vi "Motor Speed AO Message Loop.vi"(8 "error in (no error)":errorcluster, 11 "Message Queues":T1) -> (0 "error out":errorcluster)   [LabVIEW 2016, in "Motor Speed AO.lvlib"]
doc: "The message loop subVI to handle messages pertaining to logging data."
uses:
  Motor Speed AO.lvlib
  support/Message Queue/All Message Queues.ctl
  support/Message Queue/Message Cluster.ctl
  MSpeed AO State.ctl
  MSpeed_MHL Data.ctl
  MSpeed AO HW Config.ctl
  <vilib>/DAQmx/write.llb/DAQmx Write (Analog Wfm 1Chan NSamp).vi
  support/Message Queue/Enqueue Message (Single).vi
  <vilib>/DAQmx/create/channels.llb/DAQmx Create Channel (AO-Voltage-Basic).vi
  <vilib>/DAQmx/configure/timing.llb/DAQmx Timing (Sample Clock).vi
  <vilib>/DAQmx/miscellaneous.llb/DAQmx Fill In Error Info.vi
  <vilib>/Utility/error.llb/Error Cluster From Error Code.vi
  <vilib>/ErrorRing/Error Ring.xnode
  support/Message Queue/Message Queue.lvlib
  <resource>/objmgr/daqmx.rc
  <vilib>/measure/NI_MABase.lvlib
  <instrlib>/Pololu Motor Controller/Pololu Motor Controller.lvlib
panel:
  out "Actual Sample Rate":dbl=1000.0 format="%0.2f"
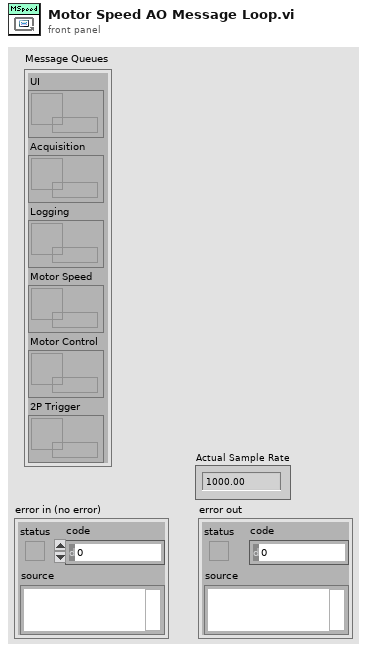
[diagram p1: front panel]
types:
  T1 = typedef "Message Queue.lvlib/All Message Queues.ctl" = cluster{"UI":refnum<queue>, "Acquisition":refnum<queue>, "Logging":refnum<queue>, "Motor Speed":refnum<queue>, "Motor Control":refnum<queue>, "2P Trigger":refnum<queue>}
  T2 = typedef "Motor Speed AO.lvlib/MSpeed AO State.ctl" = enum16{"Idle", "Running"}
  T3 = enum16{"Sine Wave", "Triangle Wave", "Square Wave", "Sawtooth Wave"}
  T4 = typedef "Motor Speed AO.lvlib/MSpeed_MHL Data.ctl" = cluster{"MSpeed HW Config":T5, "Motor VISA resource name":refnum<visa-resource-name>}
  T5 = typedef "Motor Speed AO.lvlib/MSpeed AO HW Config.ctl" = cluster{"MSpeed AO Channel":tag, "Sample Rate(Hz)":dbl, "MSpeed AO Task":refnum<k21>}
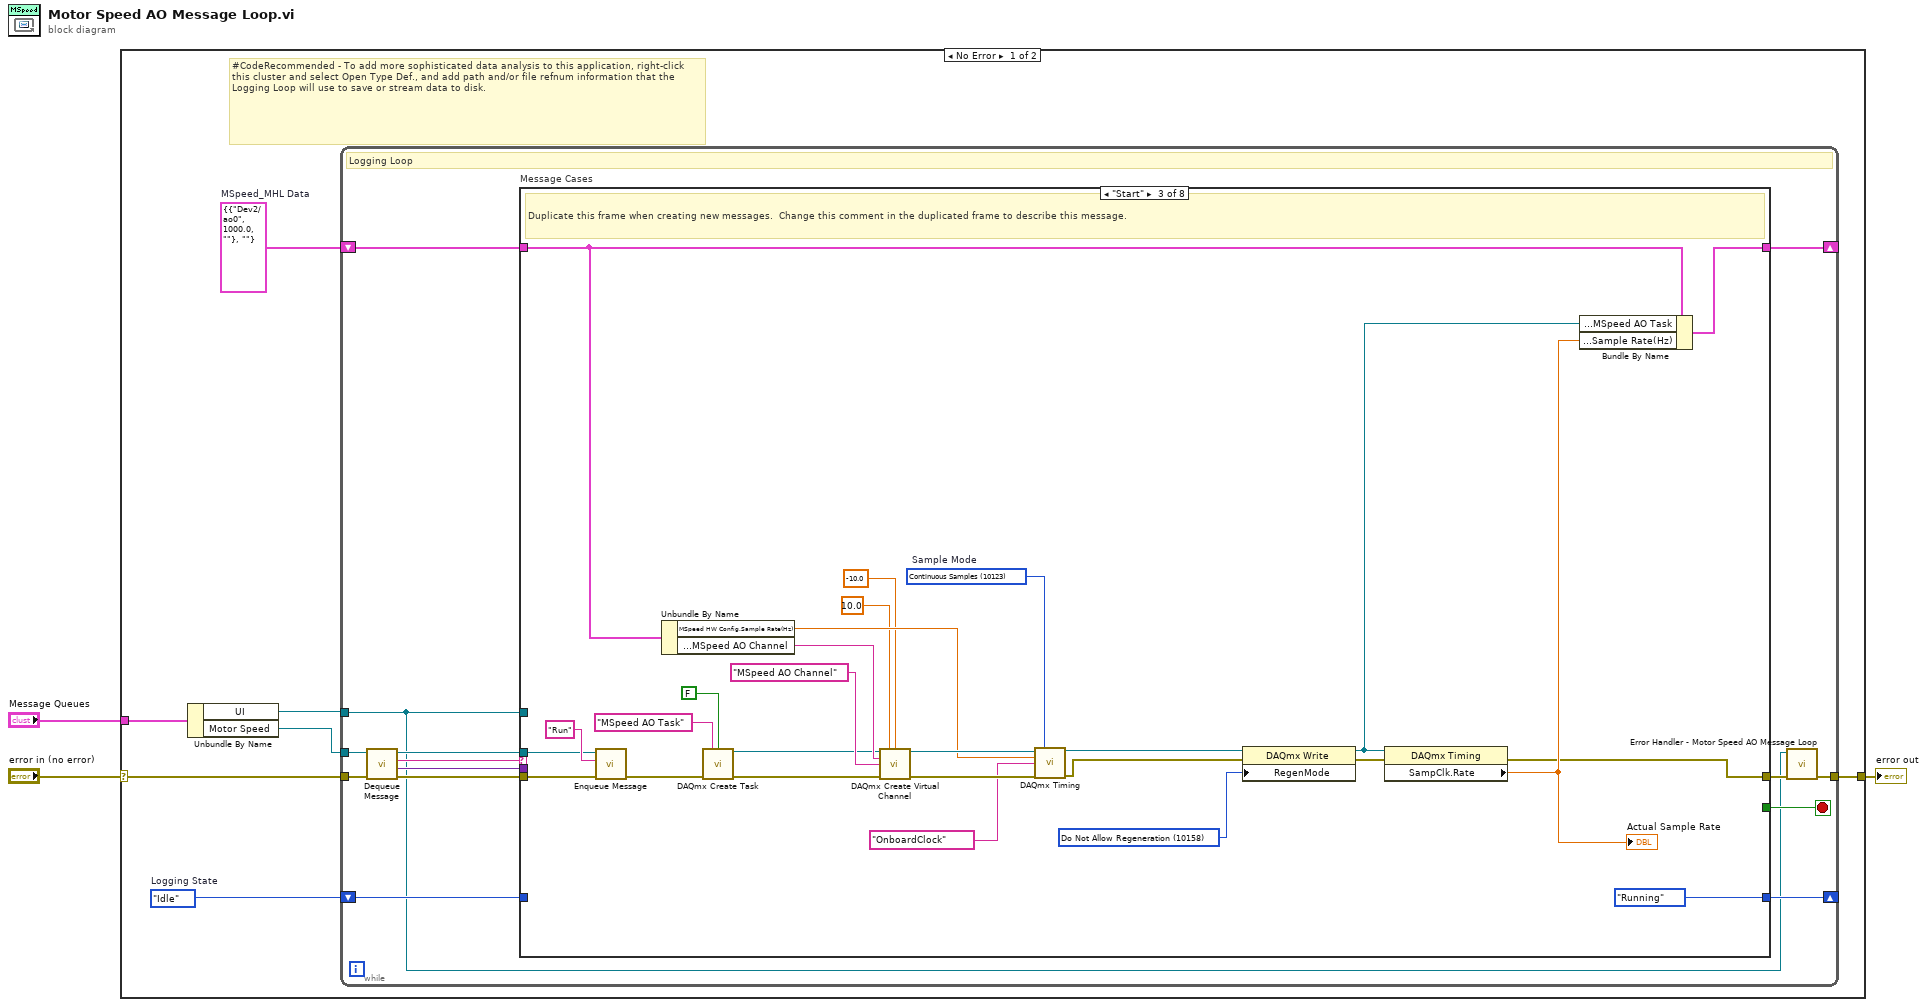
[diagram p0: block diagram]
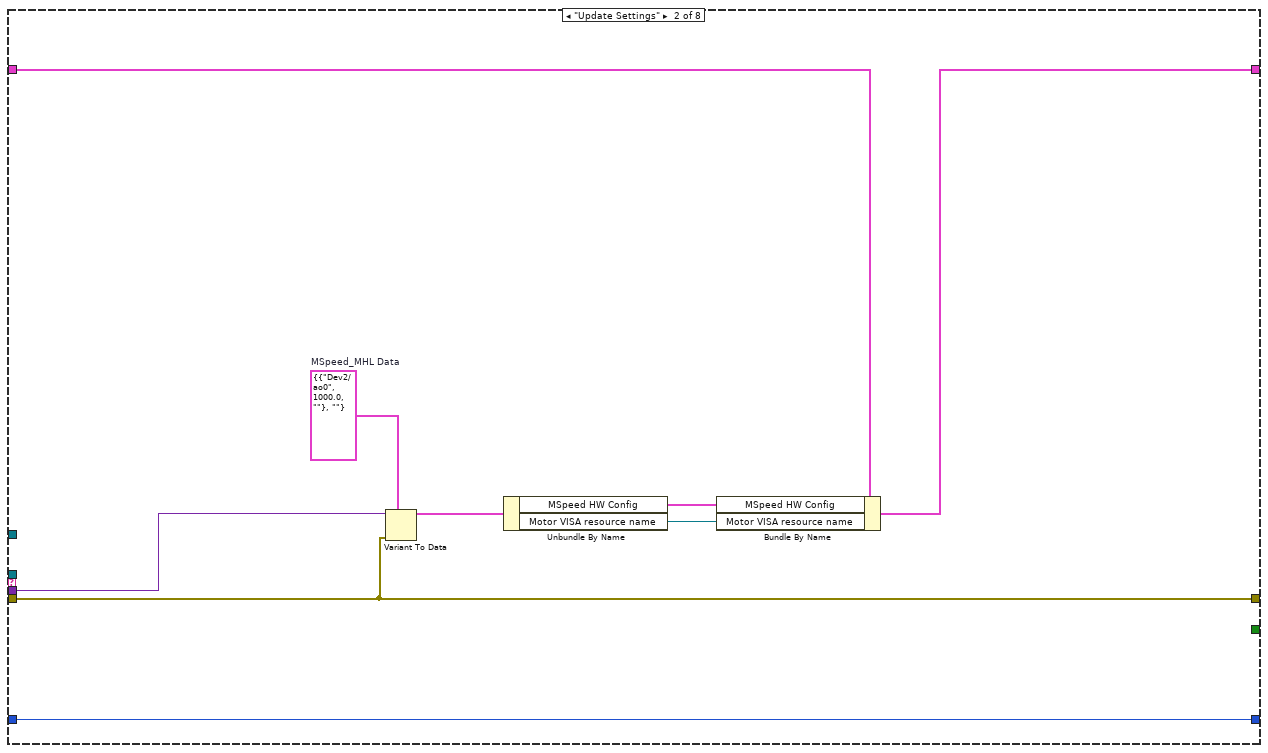
[diagram p3: hidden frame]
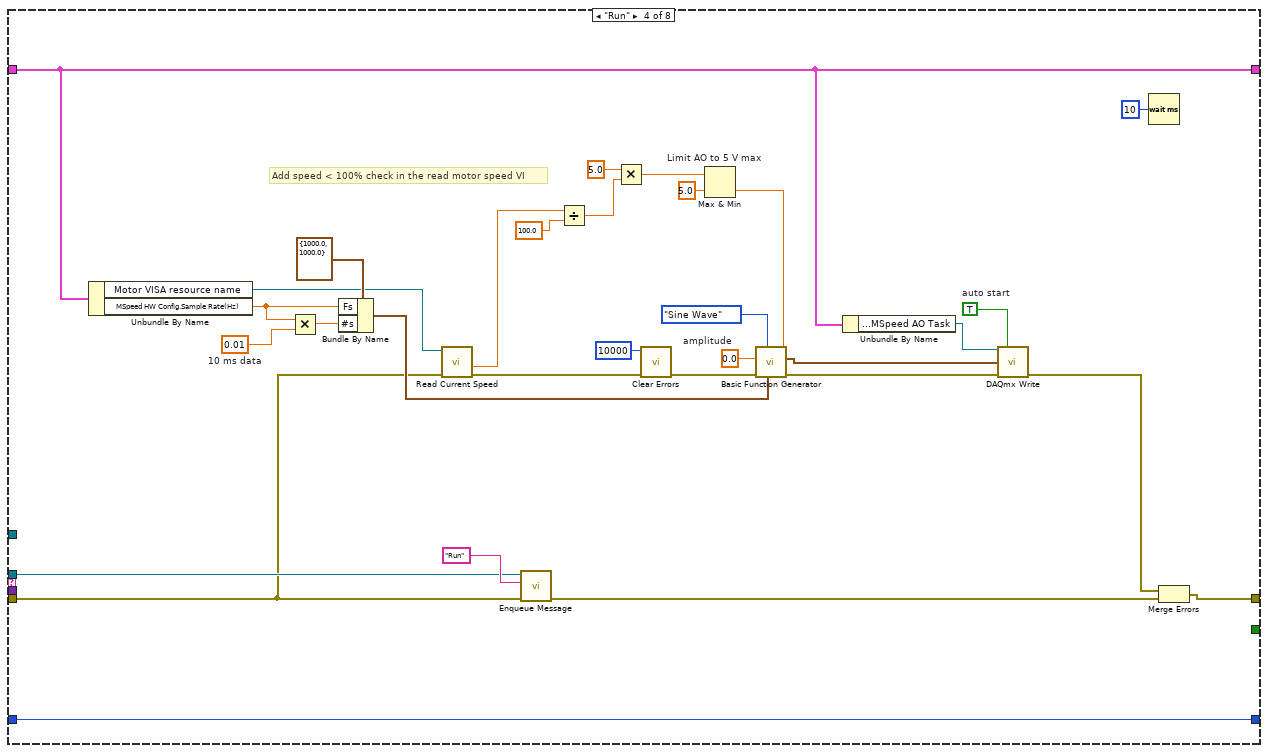
[diagram p4: hidden frame]
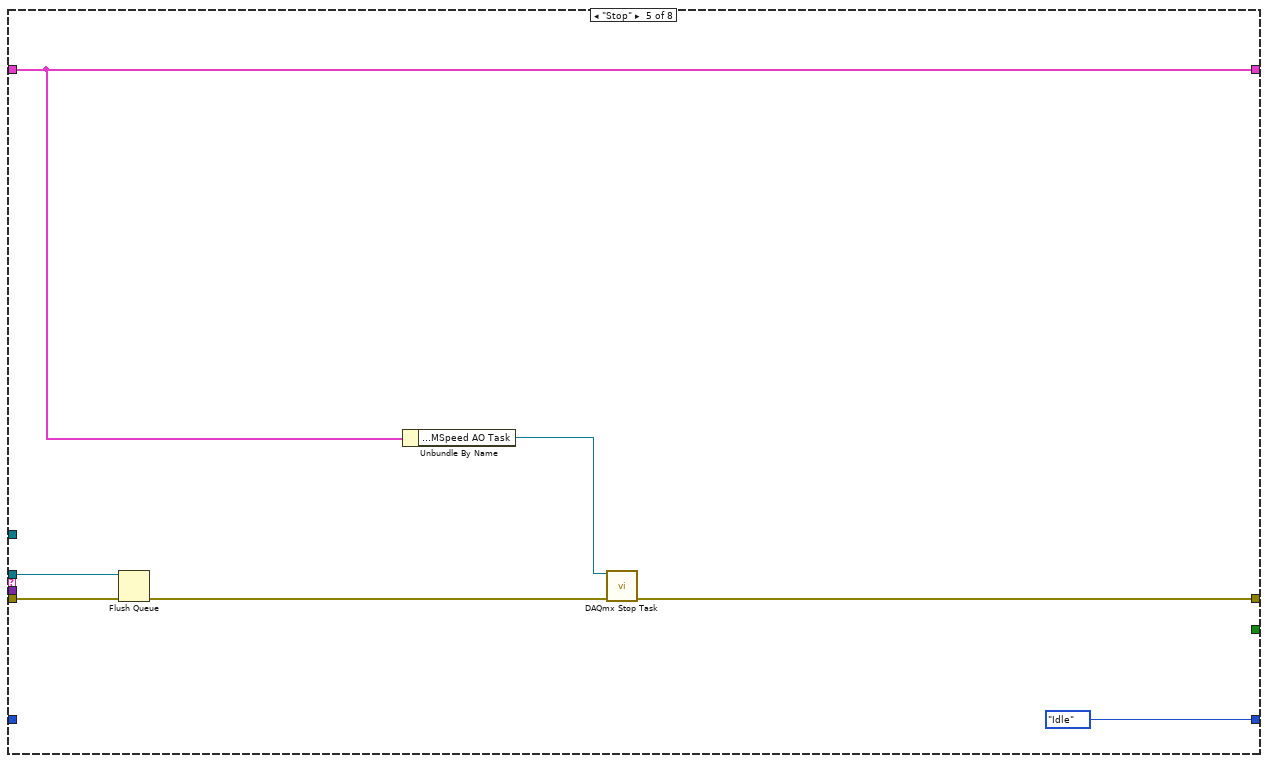
[diagram p5: hidden frame]
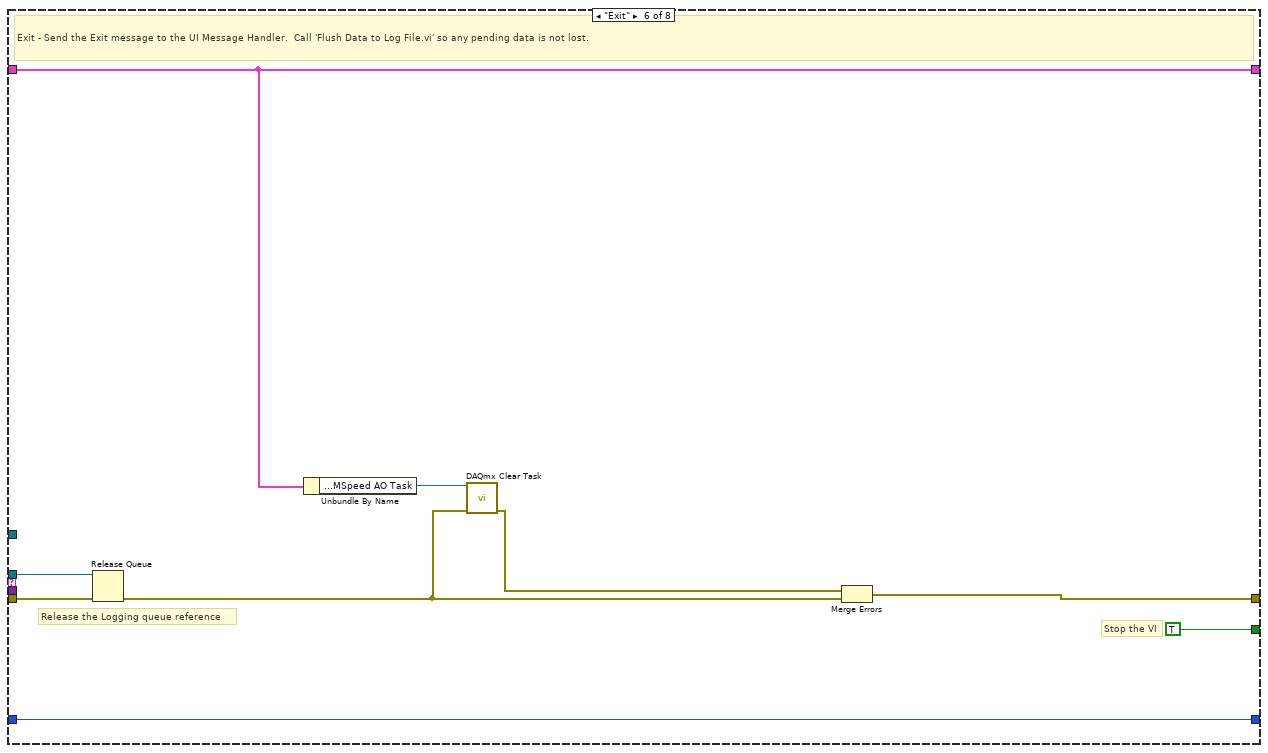
[diagram p6: hidden frame]
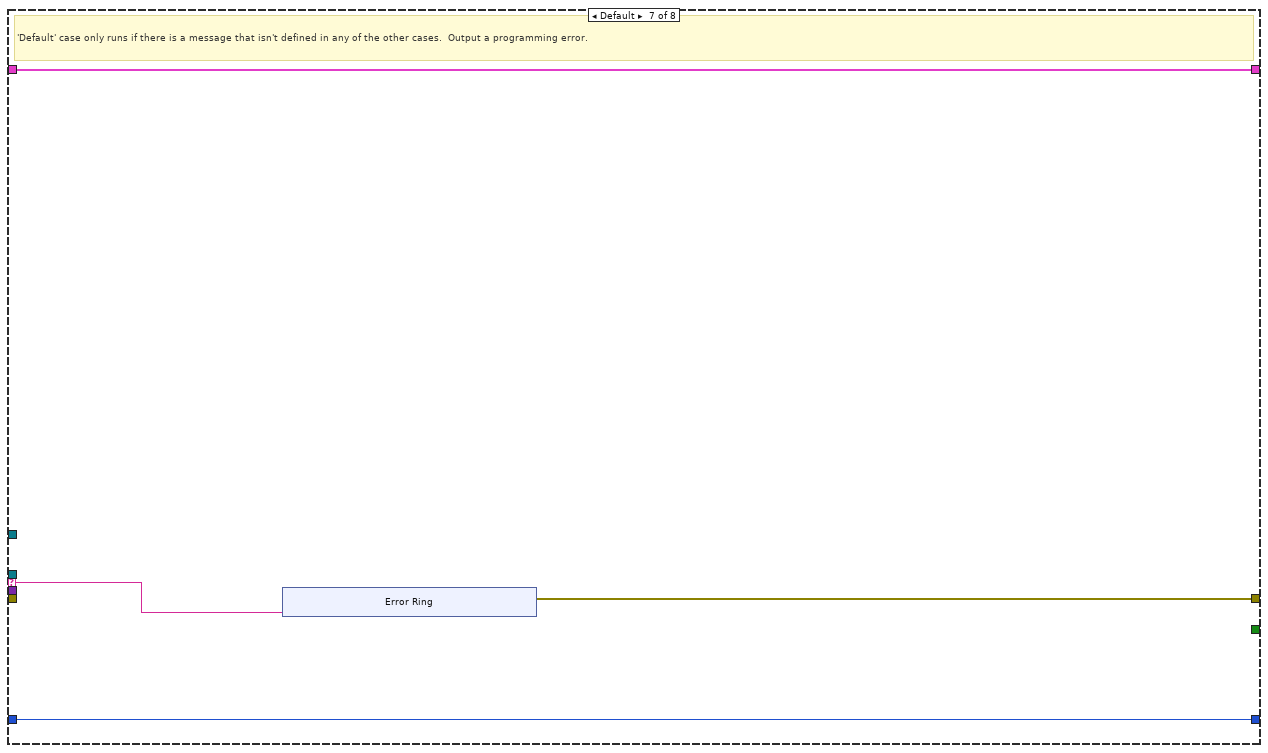
[diagram p7: hidden frame]
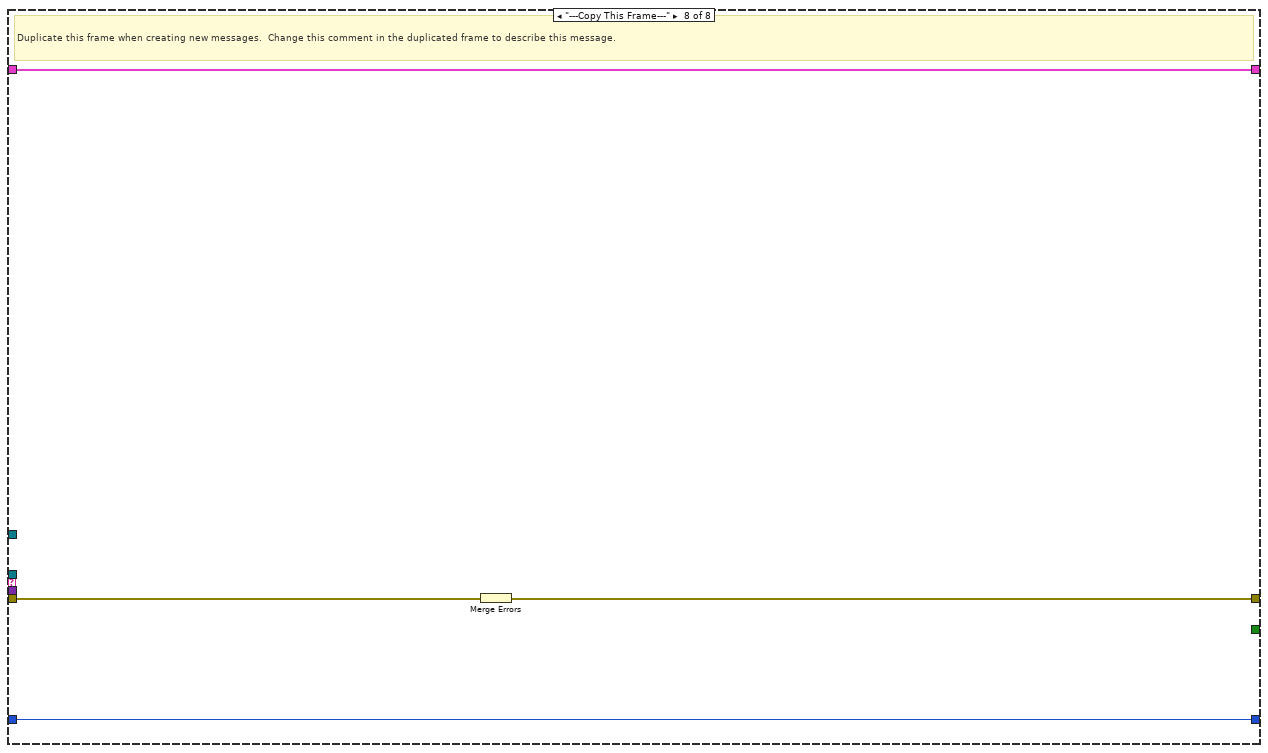
[diagram p8: hidden frame]
diagram:
  n1 = case shown="No Error" "error in (no error)" {
    selector: "error in (no error)" -> [w7 w126]
    tunnel: "Message Queues" -> [w10 _]
    tunnel: [w8 w126] -> w2
    frame No Error {
      w4 = T4 {"MSpeed HW Config"={"MSpeed AO Channel"="Dev2/ao0", "Sample Rate(Hz)"=1000.0, "MSpeed AO Task"=""}, "Motor VISA resource name"=""}  # MSpeed_MHL Data
      w5 = MSpeed_AO_State."Idle"  # Logging State
      # "#CodeRecommended - To add more sophisticated data analysis to this application, right-click this cluster and select Open Type Def., and add path and/or file refnum information that the Logging Loop will use to save or stream data to disk."
      n2 = Unbundle By Name(w10) -> ("UI"=w6:refnum<queue>, "Motor Speed"=w9:refnum<queue>)
      n3 = while {
        tunnel: w9 -> [w16]
        shift-right: [w23] -> _
        shift-left: w4 -> [w24]
        tunnel: w6 -> [w11]
        shift-right: [w14] -> _
        shift-left: w5 -> [w15]
        tunnel: w7 -> [w21]
        tunnel: [w13] -> w8
        stop <- w22 stop-if-true
        # "Logging Loop"
        n4 = call "Dequeue Message.vi"("error in (no error)"=w21, "Message Queue"=w16) -> ("error out"=w20:errorcluster, "Message Data"=w18:variant, "Message"=w19:string, "dup Message Queue"=w17:refnum<queue>)  [unwired: 6 in]
        n5 = case "Message Cases" shown="\"Start\"" w19 {
          selector: w19 -> [_ _ _ _ _ _ w111 _]
          tunnel: w17 -> [_ _ w61 w80 w96 w107 _ _]
          tunnel: w20 -> [w26 w35 w57 w75 w98 w108 _ w125]
          tunnel: [w26 w35 w37 w79 w101 w109 w112 w123] -> w12
          tunnel: w24 -> [w27 w33 w53 w86 w100 w103 w114 w124]
          tunnel: [w27 w32 w50 w86 w100 w103 w114 w124] -> w23
          tunnel: [_ _ _ _ _ TRUE _ _] -> w22
          tunnel: w18 -> [_ w34 _ _ _ _ _ _]
          tunnel: w11 -> [_ _ _ _ _ _ _ _]
          tunnel: w15 -> [w25 w36 _ w94 _ w106 w113 w122]
          tunnel: [w25 w36 MSpeed_AO_State."Running" ("Logging State") w94 MSpeed_AO_State."Idle" ("Logging State") w106 w113 w122] -> w14
          frame "Initialize" {
            # "Initialize - gets called when first launched. Currently a no-op."
          }
          frame "Update Settings" {
            w28 = T4 {"MSpeed HW Config"={"MSpeed AO Channel"="Dev2/ao0", "Sample Rate(Hz)"=1000.0, "MSpeed AO Task"=""}, "Motor VISA resource name"=""}  # MSpeed_MHL Data
            n6 = Variant To Data(error in=w35, type=w28, Variant=w34) -> (data=w29:T4)  [unwired: 1 out]
            n7 = Unbundle By Name(w29) -> ("MSpeed HW Config"=w30:T5, "Motor VISA resource name"=w31:refnum<visa-resource-name>)
            n8 = Bundle By Name(cluster=w33, "MSpeed HW Config"=w30, "Motor VISA resource name"=w31) -> (w32:T4)
          }
          frame "Start" {
            w55 = 10158 items=["Allow Regeneration"=10097, "Do Not Allow Regeneration"=10158] ("RegenMode")
            w63 = 10123 items=["Finite Samples"=10178, "Continuous Samples"=10123, "Hardware Timed Single Point"=12522]  # Sample Mode
            # "Duplicate this frame when creating new messages.  Change this comment in the duplicated frame to describe this message."
            n9 = call-poly "Enqueue Message.vi"("error in (no error)"=w57, "Message"="Run", "Message Queue"=w61) -> ("error out"=w49:errorcluster)  [unwired: 7 in, 1 out]
            n10 = Unbundle By Name(w53) -> ("MSpeed HW Config.Sample Rate(Hz)"=w41:dbl, "MSpeed HW Config.MSpeed AO Channel"=w54:tag)
            n11 = call <vilib>:"DAQmx Create Task.vi"("new task name"="MSpeed AO Task", "auto cleanup"=FALSE, "error in"=w49) -> ("task out"=w45:refnum<k21>, "error out"=w48:errorcluster)  [unwired: 11 in]
            n12 = call-poly <vilib>:"DAQmx Create Virtual Channel.vi"("task in"=w45, "maximum value"=10.0, "minimum value"=-10.0, "physical channels"=w54, "name to assign"="MSpeed AO Channel", "error in"=w48) -> ("task out"=w59:refnum<k21>, "error out"=w58:errorcluster)  [unwired: 8 in]
            n13 = call-poly <vilib>:"DAQmx Timing.vi"("task/channels in"=w59, "sample mode"=w63, "rate"=w41, "source"=tag "OnboardClock", "error in"=w58) -> ("task out"=w42:refnum<k21>, "error out"=w43:errorcluster)  [unwired: 9 in]
            n14 = property class="DAQmx Write"(reference=w42, error in=w43, "RegenMode"=w55) -> (reference out=w52:refnum<k21>, error out=w56:errorcluster)
            n15 = property class="DAQmx Timing"(reference=w52, error in=w56) -> (error out=w37:errorcluster, "SampClk.Rate"=w51:dbl)  [unwired: 1 out]
            "Actual Sample Rate" <- w51
            n16 = Bundle By Name(cluster=w53, "MSpeed HW Config.MSpeed AO Task"=w52, "MSpeed HW Config.Sample Rate(Hz)"=w51) -> (w50:T4)
          }
          frame "Run" {
            w83 = 0.01  # 10 ms data
            w88 = 0.0  # amplitude
            w93 = TRUE  # auto start
            # "Add speed < 100% check in the read motor speed VI"
            n17 = Unbundle By Name(w86) -> ("Motor VISA resource name"=w68:refnum<visa-resource-name>, "MSpeed HW Config.Sample Rate(Hz)"=w85:dbl)
            n18 = Multiply(x=w85, y=w83) -> (x*y=w84:dbl)
            n19 = Bundle By Name(cluster=cluster{"Fs":dbl, "#s":dbl} {"Fs"=1000.0, "#s"=1000.0} ("sampling info"), "Fs"=w85, "#s"=w84) -> (w82:cluster{"Fs":dbl, "#s":dbl})
            n20 = call <instrlib>:"Read Current Speed.vi"("error in (no error)"=w75, "VISA resource name"=w68) -> ("error out"=w71:errorcluster, "Motor Speed (%)"=w66:dbl)  [unwired: 6 in, 2 out]
            n21 = call-poly "Enqueue Message.vi"("error in (no error)"=w75, "Message"="Run", "Message Queue"=w80) -> ("error out"=w77:errorcluster)  [unwired: 7 in, 1 out]
            n22 = Divide(x=w66, y=100.0) -> (x/y=w73:dbl)
            n23 = Multiply(x=5.0, y=w73) -> (x*y=w64:dbl)
            n24 = call <vilib>:"Clear Errors.vi"("error in (no error)"=w71, "specific error code to clear (0: all)"=10000) -> ("error out"=w70:errorcluster)  [unwired: 4 in, 1 out]
            n25 = Max & Min "Limit AO to 5 V max"(x=w64, y=5.0) -> (min(x,y)=w65:dbl)  [unwired: 1 out]
            n26 = call <vilib>:"Basic Function Generator.vi"("offset"=w65, "sampling info"=w82, "signal type"=T3."Sine Wave", "error in (no error)"=w70, "amplitude"=w88) -> ("error out"=w91:errorcluster, "signal out"=w90:waveform(dbl))  [unwired: 4 in, 1 out]
            n27 = Unbundle By Name(w86) -> ("MSpeed HW Config.MSpeed AO Task"=w92:refnum<k21>)
            n28 = call-poly <vilib>:"DAQmx Write.vi"("task/channels in"=w92, "auto start"=w93, "data"=w90, "error in"=w91) -> ("error out"=w78:errorcluster)  [unwired: 9 in, 2 out]
            n29 = Wait (ms)(milliseconds to wait=u32 10) -> ()  [unwired: 1 out]
            n30 = Merge Errors(w78, w77) -> (w79:errorcluster)
          }
          frame "Stop" {
            n31 = Flush Queue(queue=w96, error in (no error)=w98) -> (error out=w97:errorcluster)  [unwired: 2 out]
            n32 = Unbundle By Name(w100) -> ("MSpeed HW Config.MSpeed AO Task"=w99:refnum<k21>)
            n33 = call <vilib>:"DAQmx Stop Task.vi"("task/channels in"=w99, "error in"=w97) -> ("error out"=w101:errorcluster)  [unwired: 12 in, 1 out]
          }
          frame "Exit" {
            # "Release the Logging queue reference"
            # "Stop the VI"
            # "Exit - Send the Exit message to the UI Message Handler.  Call 'Flush Data to Log File.vi' so any pending data is not lost."
            n34 = Release Queue(queue=w107, error in (no error)=w108) -> (error out=w105:errorcluster)  [unwired: 1 in, 2 out]
            n35 = Unbundle By Name(w103) -> ("MSpeed HW Config.MSpeed AO Task"=w102:refnum<k21>)
            n36 = call <vilib>:"DAQmx Clear Task.vi"("task in"=w102, "error in"=w105) -> ("error out"=w104:errorcluster)  [unwired: 13 in]
            n37 = Merge Errors(w104, w105) -> (w109:errorcluster)
          }
          frame Default {
            # "'Default' case only runs if there is a message that isn't defined in any of the other cases.  Output a programming error."
            n38 = xnode "Error Ring"("parameter 0"=w111) -> ("error out"=w112:errorcluster)
          }
          frame "---Copy This Frame---" {
            # "Duplicate this frame when creating new messages.  Change this comment in the duplicated frame to describe this message."
            n39 = Merge Errors(w125) -> (w123:errorcluster)
          }
        }
        n40 = call "Error Handler - Motor Speed AO Message Loop.vi"("error in (no error)"=w12, "Message Queue"=w11) -> ("dup error in"=w13:errorcluster)  [unwired: 8 in, 1 out]
      }
    }
    frame Error {
    }
  }
  "error out" <- w2
